vi "Lab08_Unconfigure_IMAQ.vi"(8 "error in (no error)":errorcluster, 10 "Images to dispose":T2[](array[typedef]), 11 "IMAQdx session in":T1) -> (0 "error out":errorcluster)   [LabVIEW 2021]
doc: "Unconfigures and closes the camera for DAQSP Lab05. This VI also releases the allocated frame buffers."
uses:
  <vilib>/vision/Image Controls.llb/IMAQ Image.ctl
  <vilib>/userDefined/High Color/IMAQdx.ctl
  <vilib>/vision/driver/NI_Vision_Acquisition_Software.lvlib
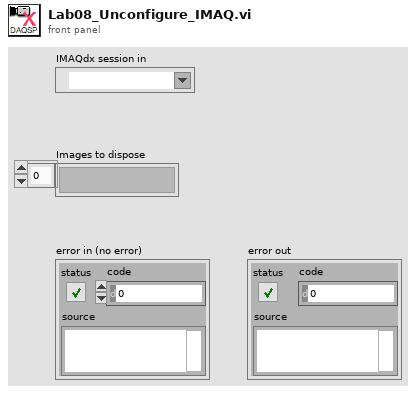
[diagram p1: front panel]
types:
  T1 = typedef "IMAQdx.ctl" = refnum<k21>
  T2 = typedef "IMAQ Image.ctl" = refnum<image>
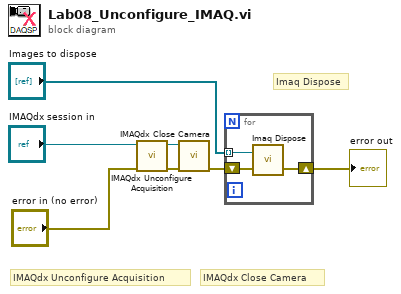
[diagram p0: block diagram]
diagram:
  # "Imaq Dispose"
  # "IMAQdx Close Camera"
  # "IMAQdx Unconfigure Acquisition"
  n1 = call <vilib>:"IMAQdx Unconfigure Acquisition.vi"("error in"="error in (no error)", "Session In"="IMAQdx session in") -> ("error out"=w2:errorcluster, "Session Out"=w1:T1)  [unwired: 8 out]
  n2 = call <vilib>:"IMAQdx Close Camera.vi"("error in"=w2, "Session In"=w1) -> ("error out"=w6:errorcluster)  [unwired: 9 out]
  n3 = for {
    shift-right: [w9] -> w5
    shift-left: w6 -> [w10]
    tunnel: "Images to dispose" -> [w8] mode=indexing
    n4 = call "Imaq Dispose"("Image"=w8, "error in (no error)"=w10) -> ("error out"=w9:errorcluster)  [unwired: 4 in]
  }
  "error out" <- w5
